vi "valor_medio.vi"(11 "Waveform_input":waveform(dbl)) -> (3 "Valor_medio":dbl)   [LabVIEW 2009]
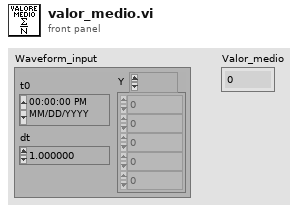
[diagram p1: front panel]
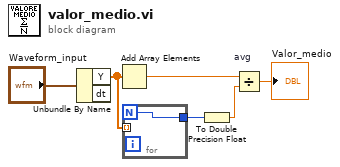
[diagram p0: block diagram]
diagram:
  n1 = Unbundle By Name("Waveform_input") -> ("Y"=w2:dbl[])  [unwired: 1 out]
  n2 = Add Array Elements(numeric array=w2) -> (sum=w3:dbl)
  n3 = for {
    N -> [w7]
    tunnel: w2 -> [_] mode=indexing
    tunnel: [w7] -> w4
  }
  n4 = To Double Precision Float(number=w4) -> (double precision float=w5:dbl)
  n5 = Divide "avg"(x=w3, y=w5) -> (x/y=→"Valor_medio":dbl)
